vi "SetOperationStatus.vi"(8 "error in":errorcluster, 10 "OperationStatus":T1=enum."NOT_COMPLETED", 11 "OperationRun in":refnum<class "OperationRun.lvclass">) -> (0 "error out":errorcluster, 3 "OperationRun out":refnum<class "OperationRun.lvclass">)   [LabVIEW 2021, in "ProligentXMLGenerator.lvlib" / "OperationRun.lvclass"]
doc: "Defines the last known status of the operation run.\n\nPASS: The execution completed successfully.\nFAIL: The execution completed and failures were detected.\nNOT_COMPLETED: The execution is not completed. It is still in progress. In that situation, the end time of the execution must be ommited.\nABORTED: The execution was aborted."
uses:
  OperationRun.lvclass
  OperationRun.lvclass/OperationRun.ctl
  Base/ExecutionStatus/Value.ctl
  Base/ExecutionStatus/ExecutionStatus.lvclass
  Base/DateTime/DateTime.lvclass
  Base/Attribute/Attribute.lvclass
  C:/Projects/proligent-xml-generator-labview/src/ProligentXMLGenerator/Base/Attribute/Attribute.lvclass
  C:/Projects/proligent-xml-generator-labview/src/ProligentXMLGenerator/Base/DateTime/DateTime.lvclass
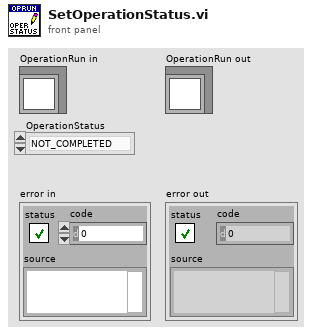
[diagram p1: front panel]
types:
  T1 = typedef "ProligentXMLGenerator.lvlib/ExecutionStatus.lvclass/Value.ctl" = enum16{"PASS", "FAIL", "NOT_COMPLETED", "ABORTED"}
  T2 = typedef "ProligentXMLGenerator.lvlib/OperationRun.lvclass/Data.ctl" = cluster{"Name":string, "Characteristics":refnum<class "Characteristic.lvclass">[], "Documents":refnum<class "Document.lvclass">[], "SequenceRuns":refnum<class "SequenceRun.lvclass">[], "FailureReferences":refnum<class "FailureReference.lvclass">[], "SequenceRunReferences":refnum<class "SequenceRunReference.lvclass">[], "CustomData":refnum<class "CustomData.lvclass">, "OperationRunId":refnum<class "Guid.lvclass">, "ProcessFullName":refnum<class "ProcessFullName.lvclass">, "ProcessVersion":refnum<class "NonEmptyString_64.lvclass">, "OperationName":refnum<class "NonEmptyString_65.lvclass">, "StationFullName":refnum<class "FullName.lvclass">, "User":refnum<class "NonEmptyString_255.lvclass">, "CallingOperationRunId":refnum<class "Guid.lvclass">, "OperationStatus":refnum<class "ExecutionStatus.lvclass">, "OperationRunStartTime":refnum<class "DateTime.lvclass">, "OperationRunEndTime":refnum<class "DateTime.lvclass">, "TimeZoneInfoId":string}
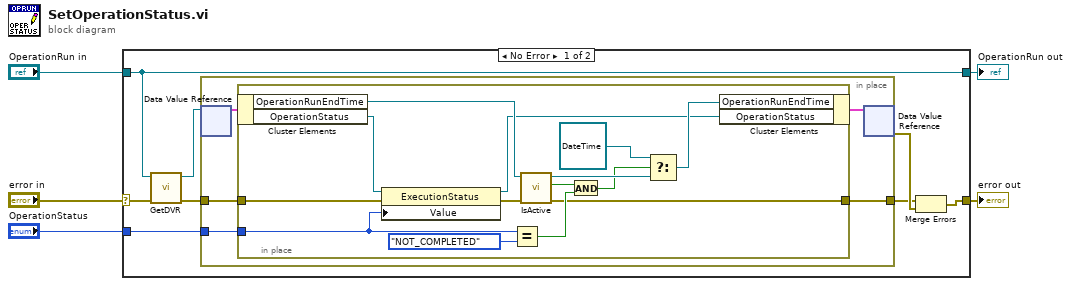
[diagram p0: block diagram]
diagram:
  n1 = case shown="No Error" "error in" {
    selector: "error in" -> [w11 w33]
    tunnel: "OperationRun in" -> [w6 w34]
    tunnel: [w8 w33] -> w3
    tunnel: "OperationStatus" -> [w7 _]
    tunnel: [w6 w34] -> w1
    frame No Error {
      n2 = call "GetDVR.vi"("error in"=w11, "OperationRun"=w6) -> ("error out"=w10:errorcluster, "DVRReference"=w12:refnum<data-value>)  [unwired: 8 in]
      n3 = in-place "In Place Element Structure" {
        in-place-border: w10 -> [w18]
        in-place-border: [w16] -> w9
        in-place-border: w7 -> [w17]
        n4 = in-place-dvr #1(w12) -> (w15:T2)  [unwired: 1 out]
        n5 = in-place "In Place Element Structure" {
          in-place-border: w18 -> [w32]
          in-place-border: w17 -> [w31]
          in-place-border: [w26] -> w16
          n6 = in-place-cluster #2(w15) -> ("OperationRunEndTime"=w22:refnum<class "DateTime.lvclass">, "OperationStatus"=w21:refnum<class "ExecutionStatus.lvclass">)
          n7 = property on="Property Node" class="ExecutionStatus"(reference=w21, error in=w32, "Value"=w31) -> (reference out=w19:refnum<class "ExecutionStatus.lvclass">, error out=w29:errorcluster)
          n8 = Equal?(x=w31, y=Value."NOT_COMPLETED") -> (x = y?=w27:bool)
          n9 = call "IsActive.vi"("error in"=w29, "Attribute in"=w22) -> ("error out"=w26:errorcluster, "IsActive"=w28:bool, "Attribute in"=w24:refnum<class "DateTime.lvclass">)  [unwired: 7 in]
          n10 = And(x=w28, y=w27) -> (x .and. y?=w23:bool)
          n11 = Select(t=refnum<class "DateTime.lvclass"> refnum ("OperationRunEndTime"), s=w23, f=w24) -> (s? t:f=w20:refnum<class "DateTime.lvclass">)
          n12 = in-place-cluster #2("OperationRunEndTime"=w20, "OperationStatus"=w19) -> (w14:T2)
        }
        n13 = in-place-dvr #1(w14) -> (w13:errorcluster)  [unwired: 1 out]
      }
      n14 = Merge Errors(w9, w13) -> (w8:errorcluster)
    }
    frame Error {
    }
  }
  "error out" <- w3
  "OperationRun out" <- w1
